vi "EMS Get Device Parameter Status.vi"(4 "Parameter/Error":string, 6 "Status":T1, 8 "error in (no error)":errorcluster, 9 "Parameter Name":string, 10 "IED Name":string, 11 "Master Controller in":refnum<class "Master Controller.lvclass">) -> (0 "error out":errorcluster, 3 "Master Controller out":refnum<class "Master Controller.lvclass">)   [LabVIEW 2015, in "Master Controller Core.lvlib" / "Master Controller.lvclass"]
uses:
  Master Controller.lvclass
  SCADA Core/SCADA Abstract Messages/Get Device Parameter Status Msg/Get Device Parameter Status.ctl
  Communications/SCADA Communcations Actor/SCADA Communications/Controls/EMS Message Cluster.ctl
  Master Controller.lvclass/Master Controller.ctl
  Communications/SCADA Communcations Actor/SCADA Communications Messages/Transmit EMS Message Msg/Transmit EMS Message Msg.lvclass/Transmit EMS Message Msg.ctl
  <vilib>/ActorFramework/Message Enqueuer/Message Enqueuer.lvclass/Message Enqueuer.ctl
  <vilib>/ActorFramework/Message Enqueuer/Enqueue.vi
  <vilib>/ActorFramework/Message Priority Queue/Priority Enqueue.vi
  Communications/SCADA Communcations Actor/SCADA Communications Messages/Transmit EMS Message Msg/Transmit EMS Message Msg.lvclass
  Utilities/Message Strings.llb/Message String Utilities.lvlib
  Communications/SCADA Communcations Actor/SCADA Communications/SCADA Communications.lvclass
  SCADA Core/SCADA Abstract Messages/Get Device Parameter Status Msg/Get Device Parameter Status Msg.lvclass
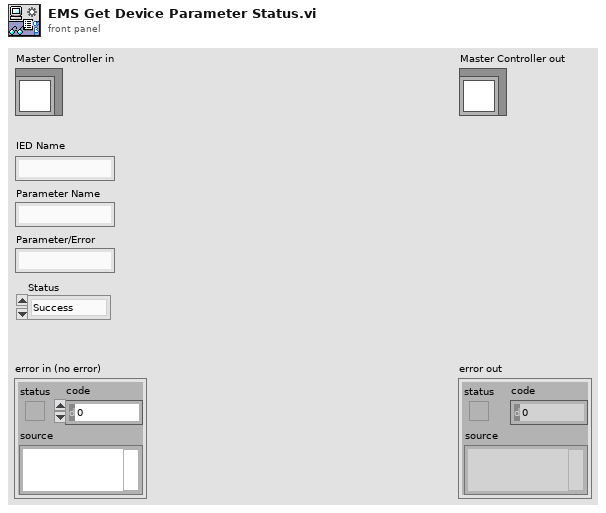
[diagram p1: front panel]
types:
  T1 = typedef "SCADA Core.lvlib/Get Device Parameter Status Msg.lvclass/Get Device Parameter Status.ctl" = enum16{"Success", "Failure"}
  T2 = typedef "SCADA Communcations Actor.lvlib/SCADA Communications.lvclass/EMS Message Cluster.ctl" = cluster{"Name":string, "Content":string}
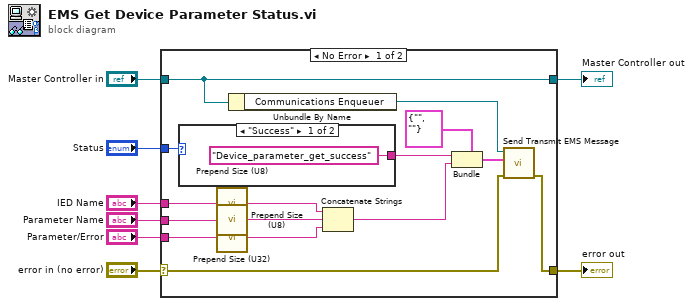
[diagram p0: block diagram]
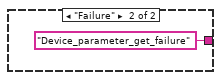
[diagram p2: hidden frame]
diagram:
  n1 = case shown="No Error" "error in (no error)" {
    selector: "error in (no error)" -> [w17 w27]
    tunnel: [w13 w27] -> w7
    tunnel: [w18 w26] -> w5
    tunnel: "Master Controller in" -> [w18 w26]
    tunnel: "Status" -> [w9 _]
    tunnel: "IED Name" -> [w16 _]
    tunnel: "Parameter Name" -> [w15 _]
    tunnel: "Parameter/Error" -> [w14 _]
    frame No Error {
      n2 = case shown="\"Success\"" w9 {
        tunnel: ["Device_parameter_get_success" ("Name") "Device_parameter_get_failure" ("Name")] -> w22
        frame "Success" {
        }
        frame "Failure" {
        }
      }
      n3 = call "Prepend Size (U8).vi"("String in"=w16) -> ("String out"=w11:string)
      n4 = call "Prepend Size (U8).vi"("String in"=w15) -> ("String out"=w12:string)
      n5 = call "Prepend Size (U32).vi"("String in"=w14) -> ("String out"=w10:string)
      n6 = Unbundle By Name(w18) -> ("Communications Enqueuer"=w20:refnum<class "Message Enqueuer.lvclass">)
      n7 = Concatenate Strings(w11, w12, w10) -> (w23:string)
      n8 = Bundle(cluster=T2 {"Name"="", "Content"=""} ("Message"), "Name"=w22, "Content"=w23) -> (w21:T2)
      n9 = call "Send Transmit EMS Message.vi"("error in (no error)"=w17, "Message"=w21, "Message Enqueuer"=w20) -> ("error out"=w13:errorcluster)  [unwired: 7 in, 1 out]
    }
    frame Error {
    }
  }
  "error out" <- w7
  "Master Controller out" <- w5
